vi "clear Session Data.vi"(0 "OBJ - Measurement Session in":refnum<class "System Log.lvclass">, 11 "error in":errorcluster) -> (4 "OBJ - Measurement Session out":refnum<class "System Log.lvclass">, 15 "error out":errorcluster)   [LabVIEW 2019, in "System Log.lvclass"]
doc: "OVERRIDE VI\nPlaceholder for decendant classes to clear session information and close references."
uses:
  System Log.lvclass
  System Log.lvclass/System Log.ctl
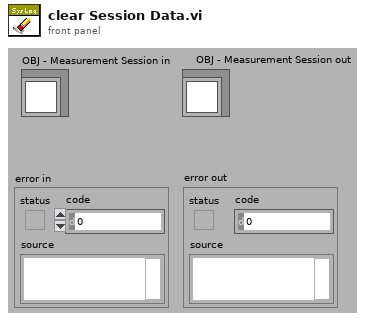
[diagram p1: front panel]
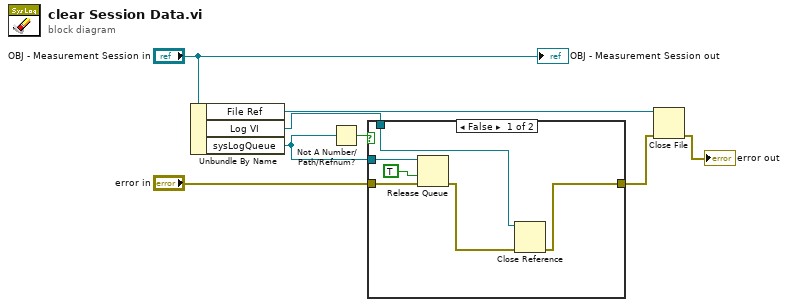
[diagram p0: block diagram]
diagram:
  n1 = Unbundle By Name("OBJ - Measurement Session in") -> ("File Ref"=w6:refnum<file>, "Log VI"=w1:refnum<vi>, "sysLogQueue"=w3:refnum<queue>)
  n2 = Not A Number/Path/Refnum?(number/path/refnum=w3) -> (NaN/Path/Refnum?=w2:bool)
  n3 = case shown="False" w2 {
    tunnel: "error in" -> [w13 w15]
    tunnel: [w10 w15] -> w5
    tunnel: w3 -> [w12 _]
    tunnel: w1 -> [w9 _]
    frame False {
      n4 = Release Queue(queue=w12, force destroy? (F)=TRUE, error in (no error)=w13) -> (error out=w11:errorcluster)  [unwired: 2 out]
      n5 = Close Reference(reference=w9, error in (no error)=w11) -> (error out=w10:errorcluster)
    }
    frame True {
    }
  }
  n6 = Close File(refnum=w6, error in=w5) -> (error out=→"error out":errorcluster)  [unwired: 1 out]
  "OBJ - Measurement Session out" <- "OBJ - Measurement Session in"
